vi "Backup_Client.vi"(1 "Check Updates on Server?":bool, 2 "Get all Server Files":bool, 3 "Months of History to backup":i32) -> (0 "error out":errorcluster)   [LabVIEW 2016]
uses:
  Anemometry/Anemometry Sub Vis/Globals/Preference_global.vi
  Anemometry/Anemometry Sub Vis/Globals/Constants_global.vi
panel:
  out "Currrently Working on":path
  out "Log of folder Done":T1(array[cluster])
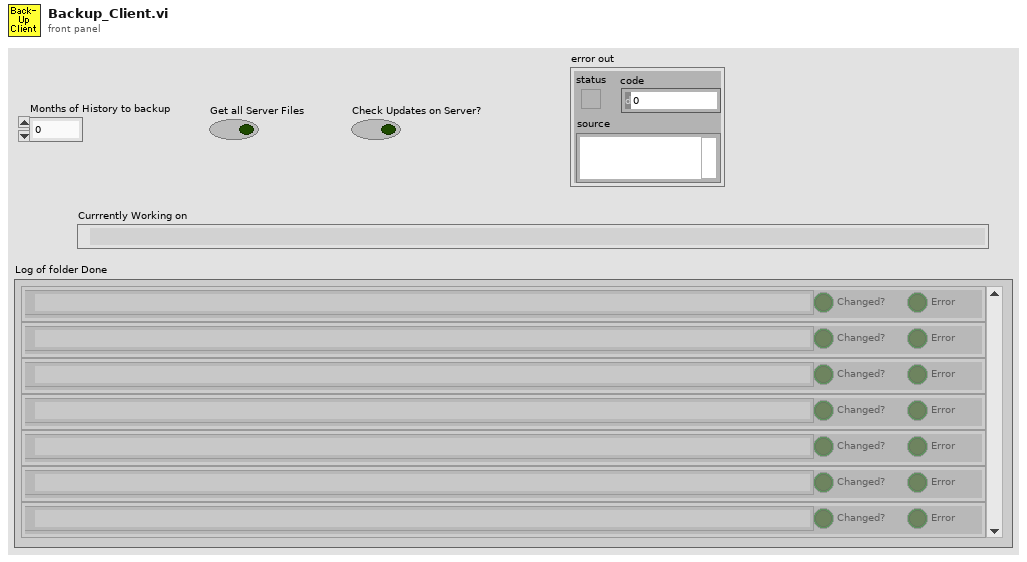
[diagram p1: front panel]
types:
  T1 = cluster{"Curnently on":path, "Changed?":bool, "Error":bool}[]
  T2 = typedef "EnFlo_Data_Folder_Setup.ctl" = string
  T3 = typedef "LVDateTimeRec.ctl" = cluster{"fractional second":dbl, "second":i32, "minute":i32, "hour":i32, "day of month":i32, "month":i32, "year":i32, "day of week":i32, "day of year":i32, "DST":i32}
  T4 = cluster{"Curnently on":path, "Changed?":bool, "Error":bool}
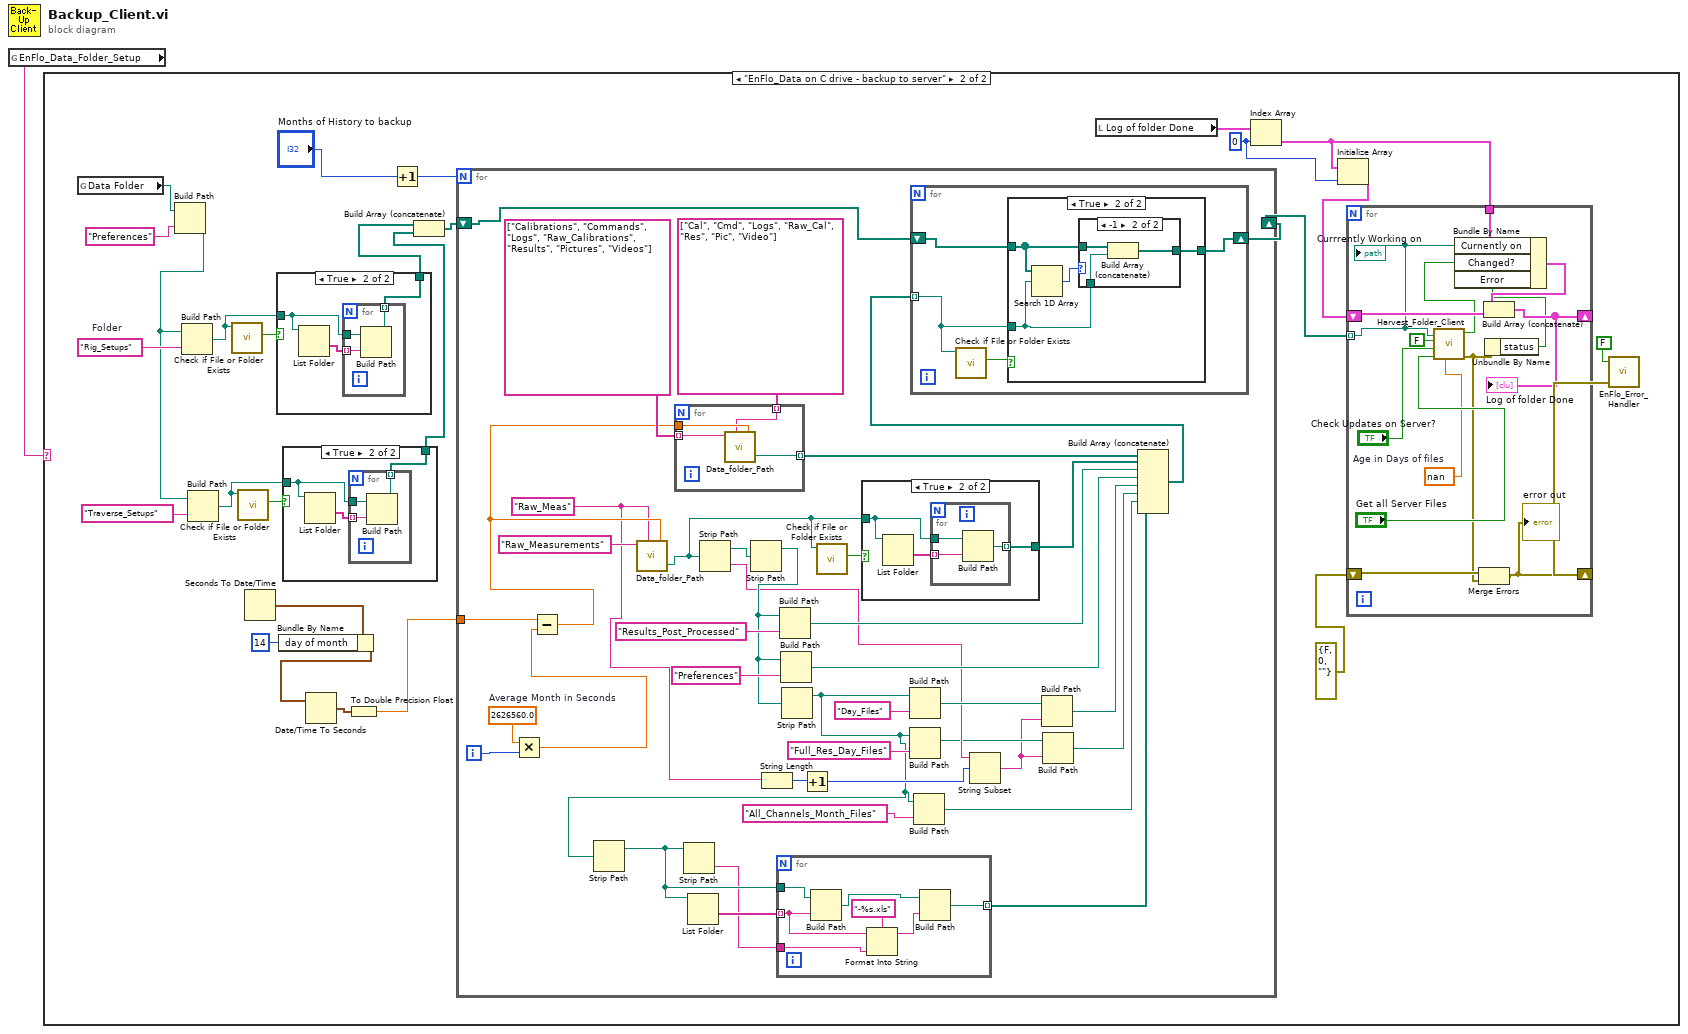
[diagram p0: block diagram]
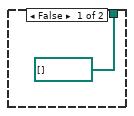
[diagram p3: hidden frame]
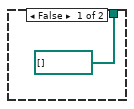
[diagram p4: hidden frame]
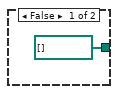
[diagram p5: hidden frame]
diagram:
  n1 = global read "Preference_global.vi" "EnFlo_Data_Folder_Setup"() -> (w1:T2)
  n2 = case shown="\"EnFlo_Data on C drive - backup to server\"" w1 {
    frame "No Match", Default {
    }
    frame "EnFlo_Data on C drive - backup to server" {
      w3 = 0 ("index")
      w12 = "Rig_Setups"  # Folder
      n3 = global read "Constants_global.vi" "Data Folder"() -> (w20:path)
      n4 = Build Path(base path=w20, name or relative path="Preferences") -> (appended path=w11:path)
      n5 = Build Path(base path=w11, name or relative path=w12) -> (appended path=w14:path)
      n6 = Build Path(base path=w11, name or relative path="Traverse_Setups") -> (appended path=w15:path)
      n7 = call <vilib>:"Check if File or Folder Exists.vi"("path"=w14) -> ("file or folder exists?"=w13:bool)  [unwired: 8 in, 2 out]
      n8 = call <vilib>:"Check if File or Folder Exists.vi"("path"=w15) -> ("file or folder exists?"=w16:bool)  [unwired: 8 in, 2 out]
      n9 = Seconds To Date/Time() -> (date time rec=w25:T3)  [unwired: 2 in]
      n10 = case shown="True" w13 {
        tunnel: [path[] [] w31] -> w9
        tunnel: w14 -> [_ w30]
        frame False {
        }
        frame True {
          n11 = List Folder(path=w30) -> (folder names=w32:string[])  [unwired: 3 in, 3 out]
          n12 = for {
            tunnel: w32 -> [w35] mode=indexing
            tunnel: w30 -> [w34]
            tunnel: [w33] -> w31 mode=indexing
            n13 = Build Path(base path=w34, name or relative path=w35) -> (appended path=w33:path)
          }
        }
      }
      n14 = Bundle By Name(cluster=w25, "day of month"=14) -> (w23:T3)
      n15 = case shown="True" w16 {
        tunnel: [path[] [] w38] -> w10
        tunnel: w15 -> [_ w37]
        frame False {
        }
        frame True {
          n16 = List Folder(path=w37) -> (folder names=w39:string[])  [unwired: 3 in, 3 out]
          n17 = for {
            tunnel: w39 -> [w42] mode=indexing
            tunnel: w37 -> [w41]
            tunnel: [w40] -> w38 mode=indexing
            n18 = Build Path(base path=w41, name or relative path=w42) -> (appended path=w40:path)
          }
        }
      }
      n19 = Date/Time To Seconds(2:w23) -> (0:w22:timestamp)  [unwired: 1 in]
      n20 = To Double Precision Float(number=w22) -> (double precision float=w26:dbl)
      n21 = Increment(x="Months of History to backup") -> (x+1=w28:i32)
      n22 = Build Array (concatenate)(w9, w10) -> (w18:path[])
      n23 = for {
        N: w28 -> [_]
        tunnel: w26 -> [w85]
        shift-right: [w80] -> w21
        shift-left: w18 -> [w81]
        i -> [w87]
        w72 = "Raw_Meas" ("Short_Name")
        w88 = 2626560.0  # Average Month in Seconds
        n24 = Multiply(x=w88, y=w87) -> (x*y=w86:dbl)
        n25 = Subtract(x=w85, y=w86) -> (x-y=w84:dbl)
        n26 = call "Data_folder_Path.vi"("Data Type"="Raw_Measurements", "Short_Name"=w72, "seconds"=w84) -> ("Data Folder"=w79:path)  [unwired: 3 in]
        n27 = for {
          tunnel: string[] ["Calibrations", "Commands", "Logs", "Raw_Calibrations", "Results", "Pictures", "Videos"] ("appended array") -> [w126] mode=indexing
          tunnel: [w125] -> w94 mode=indexing
          tunnel: w84 -> [w124]
          tunnel: string[] ["Cal", "Cmd", "Logs", "Raw_Cal", "Res", "Pic", "Video"] ("appended array") -> [w123] mode=indexing
          n28 = call "Data_folder_Path.vi"("Data Type"=w126, "Short_Name"=w123, "seconds"=w124) -> ("Data Folder"=w125:path)  [unwired: 3 in]
        }
        n29 = Strip Path(path=w79) -> (stripped path=w83:path, name=w69:string)
        n30 = Strip Path(path=w83) -> (stripped path=w76:path)  [unwired: 1 out]
        n31 = String Length(string=w72) -> (length=w71:i32)
        n32 = Build Path(base path=w76, name or relative path="Results_Post_Processed") -> (appended path=w90:path)
        n33 = Build Path(base path=w76, name or relative path="Preferences") -> (appended path=w77:path)
        n34 = Strip Path(path=w76) -> (stripped path=w61:path)  [unwired: 1 out]
        n35 = Strip Path(path=w61) -> (stripped path=w59:path)  [unwired: 1 out]
        n36 = Strip Path(path=w59) -> (name=w58:string)  [unwired: 1 out]
        n37 = List Folder(path=w59) -> (folder names=w60:string[])  [unwired: 1 in, 5 out]
        n38 = for {
          tunnel: w60 -> [w101] mode=indexing
          tunnel: w59 -> [w102]
          tunnel: w58 -> [w99]
          tunnel: [w96] -> w57 mode=indexing
          n39 = Build Path(base path=w102, name or relative path=w101) -> (appended path=w98:path)
          n40 = Format Into String(format string="-%s.xls", initial string=w101, w99) -> (resulting string=w97:string)  [unwired: 1 in, 1 out]
          n41 = Build Path(base path=w98, name or relative path=w97) -> (appended path=w96:path)
        }
        n42 = Increment(x=w71) -> (x+1=w70:i32)
        n43 = call <vilib>:"Check if File or Folder Exists.vi"("path"=w79) -> ("file or folder exists?"=w78:bool)  [unwired: 8 in, 2 out]
        n44 = case shown="True" w78 {
          tunnel: [path[] [] w105] -> w89
          tunnel: w79 -> [_ w104]
          frame False {
          }
          frame True {
            n45 = List Folder(path=w104) -> (folder names=w106:string[])  [unwired: 3 in, 3 out]
            n46 = for {
              tunnel: w106 -> [w109] mode=indexing
              tunnel: w104 -> [w108]
              tunnel: [w107] -> w105 mode=indexing
              n47 = Build Path(base path=w108, name or relative path=w109) -> (appended path=w107:path)
            }
          }
        }
        n48 = Build Path(base path=w61, name or relative path="Day_Files") -> (appended path=w74:path)
        n49 = Build Path(base path=w61, name or relative path="Full_Res_Day_Files") -> (appended path=w66:path)
        n50 = Build Path(base path=w61, name or relative path="All_Channels_Month_Files") -> (appended path=w62:path)
        n51 = String Subset(string=w69, offset (0)=w70) -> (substring=w65:string)  [unwired: 1 in]
        n52 = Build Path(base path=w74, name or relative path=w65) -> (appended path=w67:path)
        n53 = Build Path(base path=w66, name or relative path=w65) -> (appended path=w64:path)
        n54 = Build Array (concatenate)(w94, w89, w90, w77, w67, w64, w62, w57) -> (w82:path[])
        n55 = for {
          shift-right: [w112] -> w80
          shift-left: w81 -> [w113]
          tunnel: w82 -> [w111] mode=indexing
          n56 = call <vilib>:"Check if File or Folder Exists.vi"("path"=w111) -> ("file or folder exists?"=w110:bool)  [unwired: 8 in, 2 out]
          n57 = case shown="True" w110 {
            tunnel: w113 -> [w114 w117]
            tunnel: w111 -> [_ w116]
            tunnel: [w114 w118] -> w112
            frame False {
            }
            frame True {
              n58 = Search 1D Array(1D array=w117, element=w116) -> (index of element=w115:i32)  [unwired: 1 in]
              n59 = case shown="-1" w115 {
                tunnel: w117 -> [w119 w122]
                tunnel: [w119 w121] -> w118
                tunnel: w116 -> [_ w120]
                frame 0, Default {
                }
                frame -1 {
                  n60 = Build Array (concatenate)(w122, w120) -> (w121:path[])
                }
              }
            }
          }
        }
      }
      n61 = local read "Log of folder Done"() -> (w5:T1)
      n62 = Index Array(array=w5, index=w3) -> (element=w4:T4)
      n63 = Initialize Array(w4, w3) -> (w2:T1)
      n64 = for {
        tunnel: w21 -> [w49] mode=indexing
        shift-right: [w47] -> w6
        shift-left: errorcluster {"status"=FALSE, "code"=0, "source"=""} ("error constant") -> [w53]
        shift-right: [w46] -> _
        shift-left: w2 -> [w52]
        tunnel: w4 -> [w51]
        w43 = nan  # Age in Days of files
        n65 = call "Harvest_Folder_Client.vi"("Age in Days of files"=w43, "Get all Server Files"="Get all Server Files", "Check Updates on Server?"="Check Updates on Server?", "Archive Files?"=FALSE, "Folder to Harvest"=w49) -> ("error out"=w45:errorcluster, "Folder contents changed?"=w50:bool)  [unwired: 2 out]
        n66 = Merge Errors(w53, w45) -> (w47:errorcluster)
        "error out" <- w47
        n67 = Unbundle By Name(w45) -> ("status"=w44:bool)
        n68 = Bundle By Name(cluster=w51, "Curnently on"=w49, "Changed?"=w50, "Error"=w44) -> (w48:T4)
        n69 = Build Array (concatenate)(w48, w52) -> (w46:T1)
        "Log of folder Done" <- w46
        "Currrently Working on" <- w49
      }
      n70 = call "EnFlo_Error_Handler.vi"("error in (no error)"=w6, "Dialog Box (T)"=FALSE) -> ()  [unwired: 1 in, 3 out]
    }
  }
